vi "Get Channels From Expression String.vi"(8 "error in (no error)":errorcluster, 11 "Expression String in":string) -> (0 "error out":errorcluster, 1 "Channels (with quotes)":string[](array[string]), 2 "Channels":string[](array[string]), 3 "Expression String out":string)   [LabVIEW 2020, in "Output Sequencer.lvlib" / "Output Sequencer.lvclass"]
uses:
  Output Sequencer.lvclass
  7d775a17-c6d4-439b-8830-a59449ce8b25.vi
  2ab3e2e0-22f1-4255-9bcc-1ff9f547a236.vi
  <vilib>/regexp/Match Regular Expression.xnode
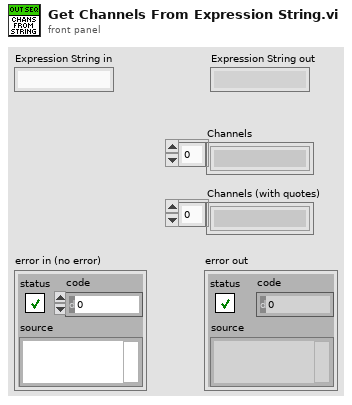
[diagram p1: front panel]
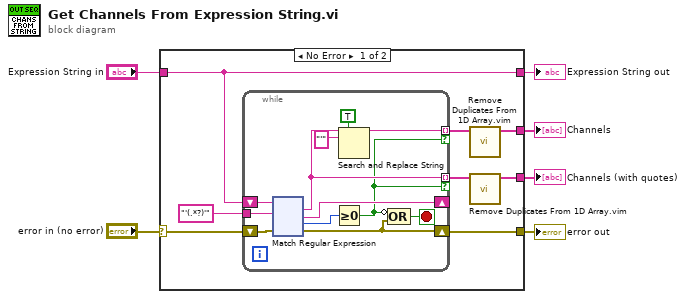
[diagram p0: block diagram]
diagram:
  n1 = case shown="No Error" "error in (no error)" {
    selector: "error in (no error)" -> [w8 w145]
    tunnel: "Expression String in" -> [w7 w144]
    tunnel: [w12 _] -> w5
    tunnel: [w11 _] -> w4
    tunnel: [w10 w145] -> w3
    tunnel: [w7 w144] -> w1
    frame No Error {
      n2 = while {
        tunnel: [w21] -> w14 mode=indexing if=w16
        shift-right: [w24] -> _
        shift-left: w7 -> [w25]
        tunnel: [w20] -> w13 mode=indexing if=w16
        shift-right: [w17] -> w10
        shift-left: w8 -> [w19]
        tunnel: "'(.*?)'" ("regular expression") -> [w18]
        stop <- w15 stop-if-true
        n3 = xnode "Match Regular Expression"("input string"=w25, "regular expression"=w18, "error in"=w19) -> ("whole match"=w21:string, "after match"=w24:string, "offset past match"=w26:i32, "error out"=w17:errorcluster)  [unwired: 3 in, 1 out]
        n4 = Greater Or Equal To 0?(x=w26) -> (x >= 0?=w16:bool)
        n5 = Search and Replace String(replace all?=TRUE ("replace all? (F)"), input string=w21, search string="'") -> (result string=w20:string)  [unwired: 5 in, 3 out]
        n6 = Compound Arithmetic op=OR(invert w16, w17) -> (w15:bool)
      }
      n7 = call "Remove Duplicates From 1D Array.vim"("array"=w13) -> ("array with duplicates removed"=w12:string[])  [unwired: 10 in]
      n8 = call "Remove Duplicates From 1D Array.vim"("array"=w14) -> ("array with duplicates removed"=w11:string[])  [unwired: 10 in]
    }
    frame Error {
    }
  }
  "Channels" <- w5
  "Channels (with quotes)" <- w4
  "Expression String out" <- w1
  "error out" <- w3
